vi "Reconfigure.vi"(8 "error in (no error)":errorcluster, 11 "TDCManager":T1) -> (0 "error out":errorcluster, 3 "TDCManager":T1)   [LabVIEW 2016, in "HPTDC Driver Library.lvlib"]
uses:
  HPTDC Driver Library.lvlib
  Typedefs/TDCManager.ctl
  C:/Users/CRT Controller/CRTC Labview Application/Source/HPTDC Driver Library Folder/Library files/hptdc_net4_3.7.0_x64.dll
  hptdc_net4_3.7.0_x64.dll
panel:
  out "Success?":bool=TRUE
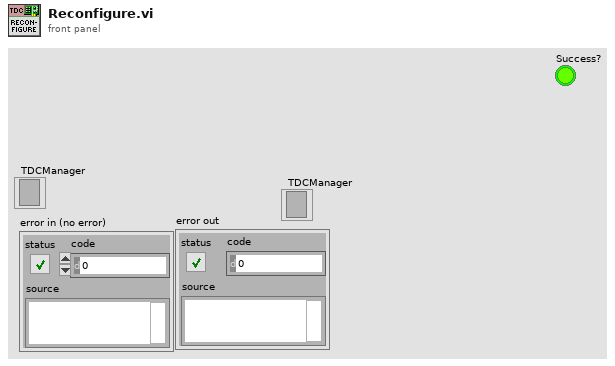
[diagram p1: front panel]
types:
  T1 = typedef "HPTDC Driver Library.lvlib/TDCManager.ctl" = refnum<k24>
  T2 = typedef "Semaphore RefNum" = refnum<k1>
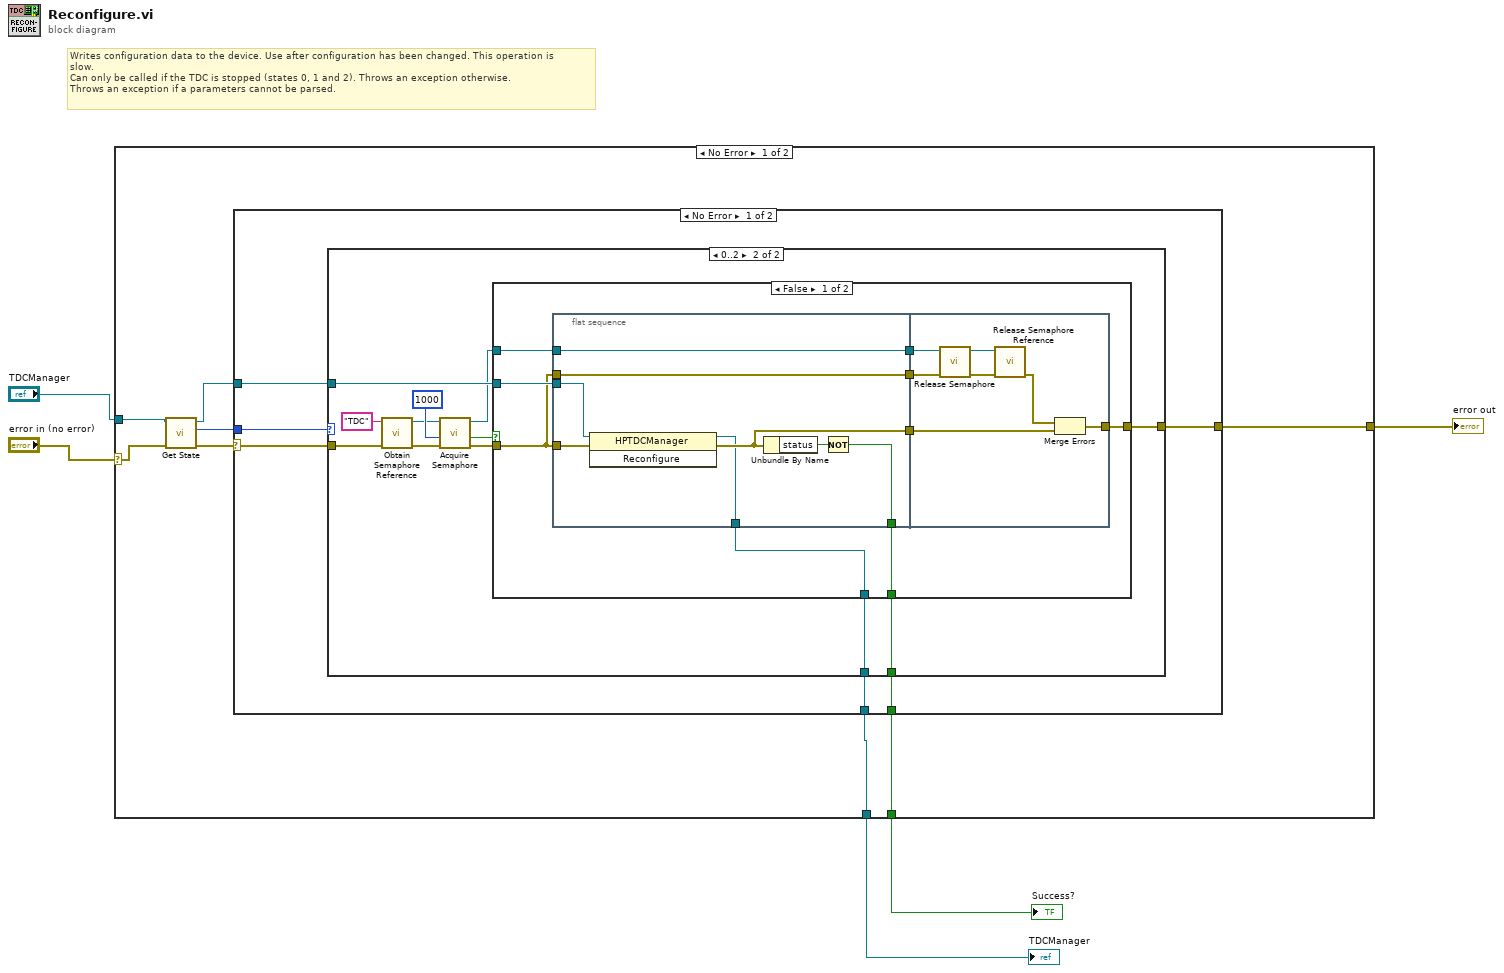
[diagram p0: block diagram]
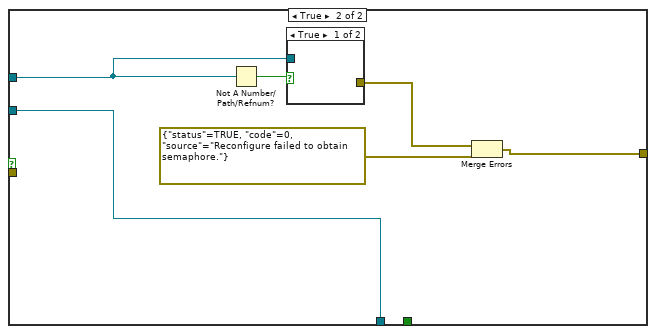
[diagram p3: hidden frame]
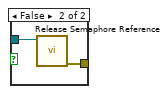
[diagram p4: hidden frame]
diagram:
  # "Writes configuration data to the device. Use after configuration has been changed. This operation is\nslow.\nCan only be called if the TDC is stopped (states 0, 1 and 2). Throws an exception otherwise.\nThrows an exception if a parameters cannot be parsed."
  n1 = case shown="No Error" "error in (no error)" {
    selector: "error in (no error)" -> [w6 w67]
    tunnel: "TDCManager" -> [w13 w68]
    tunnel: [w10 w67] -> w4
    tunnel: [w8 _] -> w3
    tunnel: [w9 w68] -> w1
    frame No Error {
      n2 = call "Get State.vi"("error in"=w6, "TDCManager"=w13) -> ("error out"=w7:errorcluster, "State"=w11:i32, "TDCManager"=w12:T1)  [unwired: 6 in, 1 out]
      n3 = case shown="No Error" w7 {
        selector: w7 -> [w14 w66]
        tunnel: w12 -> [w19 _]
        tunnel: w11 -> [w18 _]
        tunnel: [w17 w66] -> w10
        tunnel: [w16 _] -> w9
        tunnel: [w15 _] -> w8
        frame No Error {
          n4 = case shown="0..2" w18 {
            tunnel: w14 -> [w21 w28]
            tunnel: w19 -> [w20 w33]
            tunnel: [_ w24] -> w15
            tunnel: [w20 w23] -> w16
            tunnel: [w21 w22] -> w17
            frame Default {
            }
            frame 0..2 {
              n5 = call <vilib>:"Obtain Semaphore Reference.vi"("error in (no error)"=w28, "name (unnamed)"="TDC") -> ("error out"=w30:errorcluster, "semaphore"=w31:T2)  [unwired: 3 in, 1 out]
              n6 = call <vilib>:"Acquire Semaphore.vi"("error in (no error)"=w30, "ms timeout (-1)"=1000, "semaphore"=w31) -> ("error out"=w26:errorcluster, "timed out"=w27:bool, "semaphore out"=w25:T2)  [unwired: 2 in]
              n7 = case shown="False" w27 {
                tunnel: w33 -> [w42 w59]
                tunnel: w26 -> [w39 _]
                tunnel: w25 -> [w37 w58]
                tunnel: [w36 _] -> w24
                tunnel: [w35 w59] -> w23
                tunnel: [w34 w60] -> w22
                frame False {
                  n8 = flat-sequence {
                    tunnel: w39 -> [w50]
                    tunnel: w42 -> [w44]
                    tunnel: [w49] -> w41
                    tunnel: w39 -> [w47]
                    tunnel: [w47] -> w40
                    tunnel: [w46] -> w38
                    tunnel: w37 -> [w46]
                    tunnel: [w43] -> w36
                    tunnel: [w45] -> w35
                    tunnel: w41 -> [w57]
                    tunnel: w40 -> [w54]
                    tunnel: w38 -> [w52]
                    tunnel: [w51] -> w34
                    frame #0 {
                      n9 = invoke class="HPTDCManager" method="Reconfigure"(reference=w44, error in=w50) -> (reference out=w45:T1, error out=w49:errorcluster)  [unwired: 1 in, 1 out]
                      n10 = Unbundle By Name(w49) -> ("status"=w48:bool)
                      n11 = Not(x=w48) -> (.not. x?=w43:bool)
                    }
                    frame #1 {
                      n12 = call <vilib>:"Release Semaphore.vi"("error in (no error)"=w54, "semaphore"=w52) -> ("error out"=w55:errorcluster, "semaphore out"=w56:T2)  [unwired: 4 in]
                      n13 = call <vilib>:"Release Semaphore Reference.vi"("error in (no error)"=w55, "semaphore"=w56) -> ("error out"=w53:errorcluster)  [unwired: 8 in, 1 out]
                      n14 = Merge Errors(w53, w57) -> (w51:errorcluster)
                    }
                  }
                }
                frame True {
                  n15 = Not A Number/Path/Refnum?(number/path/refnum=w58) -> (NaN/Path/Refnum?=w63:bool)
                  n16 = case shown="True" w63 {
                    tunnel: [_ w65] -> w62
                    tunnel: w58 -> [_ w64]
                    frame True {
                    }
                    frame False {
                      n17 = call <vilib>:"Release Semaphore Reference.vi"("semaphore"=w64) -> ("error out"=w65:errorcluster)  [unwired: 9 in, 1 out]
                    }
                  }
                  n18 = Merge Errors(w62, errorcluster {"status"=TRUE, "code"=0, "source"="Reconfigure failed to obtain semaphore."} ("error out")) -> (w60:errorcluster)
                }
              }
            }
          }
        }
        frame Error {
        }
      }
    }
    frame Error {
    }
  }
  "error out" <- w4
  "TDCManager" <- w1
  "Success?" <- w3
